vi "newGame.vi"(8 "error in (no error)":errorcluster, 9 "playerName":string, 10 "ledRefnums":refnum<vi>[](array[refnum]), 11 "Simon_Game in":refnum<class "Simon_Game.lvclass">) -> (0 "error out":errorcluster, 3 "Simon_Game out":refnum<class "Simon_Game.lvclass">)   [LabVIEW 2019, in "Simon_Game.lvclass"]
uses:
  Simon_Game.lvclass
  Simon_Engine/Simon_Engine.lvclass
  Player/Player.lvclass
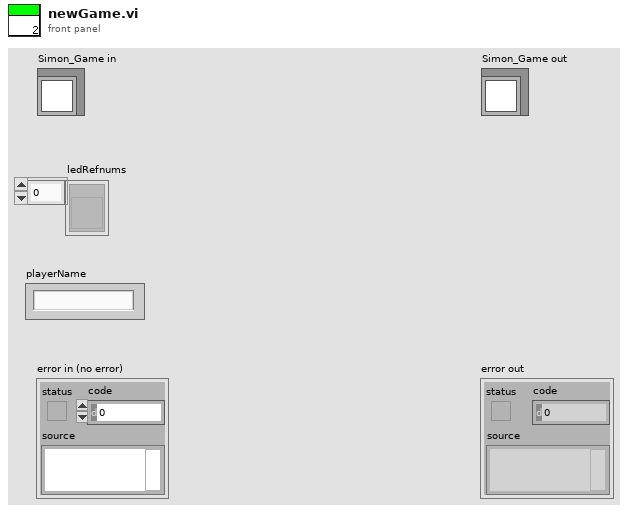
[diagram p1: front panel]
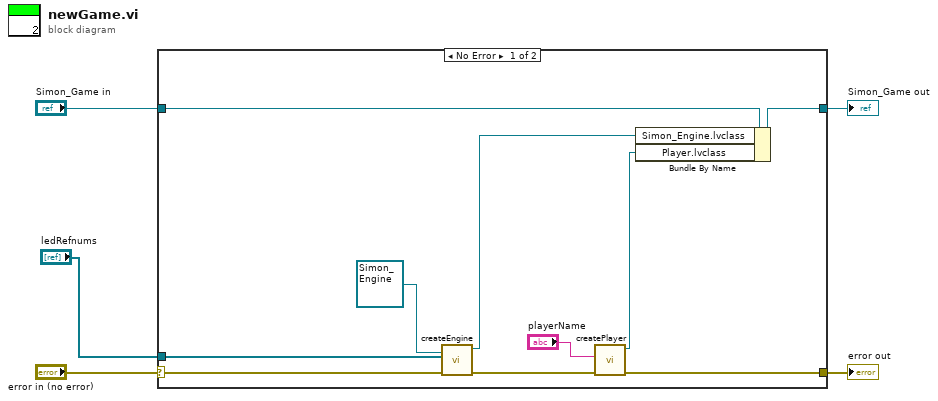
[diagram p0: block diagram]
diagram:
  n1 = case shown="No Error" "error in (no error)" {
    selector: "error in (no error)" -> [w15 w17]
    tunnel: [w8 w17] -> w4
    tunnel: [w13 w16] -> w2
    tunnel: "Simon_Game in" -> [w14 w16]
    tunnel: "ledRefnums" -> [w9 _]
    frame No Error {
      n2 = call-dynamic "createEngine.vi"(7:refnum<class "Simon_Engine.lvclass"> refnum ("Simon_Engine in"), "error in (no error)"=w15, "ledRefnums"=w9) -> ("error out"=w12:errorcluster, "Simon_Engine out"=w11:refnum<class "Simon_Engine.lvclass">)  [unwired: 7 in]
      n3 = call "createPlayer.vi"("error in (no error)"=w12, 10:"playerName") -> ("error out"=w8:errorcluster, "Player out"=w6:refnum<class "Player.lvclass">)  [unwired: 8 in]
      n4 = Bundle By Name(cluster=w14, "Simon_Engine.lvclass"=w11, "Player.lvclass"=w6) -> (w13:refnum<class "Simon_Game.lvclass">)
    }
    frame Error {
    }
  }
  "error out" <- w4
  "Simon_Game out" <- w2
